vi "Start.vi"(6 "url (\"/mcp/server\")":string="/mcp/server", 8 "error in (no error)":errorcluster, 9 "HTTP Port (36987)":u16=36987, 10 "Description":string, 11 "Name":string) -> (0 "error out":errorcluster, 2 "MCP Events":T1, 3 "server id out":i32)   [LabVIEW 2020, in "MCP Server.lvlib"]
doc: "Creates a new MCP server. The URL will be:\nhttp://localhost:3687/mcp/server\nServer name and description will be passed on to the client and the LLM. Be aware that these cost you tokes. For detailled descriptions of the server (e.g. software manual) use resources instead. \nThis VI returns user events for different events that can happen inside the server. Make sure to listen to the error event to catch any runtime errors. Use the onRpc event to receive every request that is sent from a client to the server.\n\nYour MCP Client config (e.g. claude_desktop_config.json) should look like this:\n{\n \"mcpServers\": {\n \"My Cool Server Display-Name\": {\n \"command\": \"npx\",\n \"args\": [\n \"mcp-remote\",\n \"http://127.0.0.1:36987/mcp/server\"\n ],\n \"env\": {\n \"YOUR_API_KEY\": \"<YOUR_SECRET_KEY>\",\n \"MY_PARAM\": \"Your custom Parameter\"\n }\n }\n }\n}"
uses:
  MCP Server.lvlib
  User Events.ctl
  onRpc.ctl
  Server Data.ctl
  <vilib>/IlluminatedG/IG HTTP Server/HTTP Server/server/Server.lvclass
  Tool Data.ctl
  Input Parameter.ctl
  Output Parameter.ctl
  Logging.ctl
  Prompt Data.ctl
  Prompt Argument.ctl
  resource data.ctl
  MCP Handler/MCP Handler.lvclass
  C:/Program Files/National Instruments/LabVIEW 2026/vi.lib/IlluminatedG/IG HTTP Server/HTTP Server/Handler/Handler.lvclass
  <vilib>/IlluminatedG/IG HTTP Server/HTTP Server/Server/Add Connection Handler.vi
  <vilib>/IlluminatedG/IG HTTP Server/HTTP Server/Server/Add Request Handler.vi
  <vilib>/IlluminatedG/IG HTTP Server/HTTP Server/Server/Add Route Handler.vi
  <vilib>/IlluminatedG/IG HTTP Server/HTTP Server/Server/Add Controller Handler.vi
  <vilib>/IlluminatedG/IG HTTP Server/HTTP Server/Server/Add Controller.vi
  <vilib>/IlluminatedG/IG HTTP Server/HTTP Server/Server/Add Response Handler.vi
  <vilib>/IlluminatedG/IG HTTP Server/HTTP Server/Server/Add Complete Handler.vi
  <vilib>/IlluminatedG/IG HTTP Server/HTTP Server/Server/Add Exception Handler.vi
  <vilib>/IlluminatedG/IG HTTP Server/HTTP Server/Connection Handler/Connection Handler.lvclass
  <vilib>/IlluminatedG/IG HTTP Server/HTTP Server/Request Handler/Request Handler.lvclass
  <vilib>/IlluminatedG/IG HTTP Server/HTTP Server/Route Handler/Route Handler.lvclass
  <vilib>/IlluminatedG/IG HTTP Server/HTTP Server/Controller Handler/Controller Handler.lvclass
  <vilib>/IlluminatedG/IG HTTP Server/HTTP Server/Controller/Controller.lvclass
  <vilib>/IlluminatedG/IG HTTP Server/HTTP Server/Response Handler/Response Handler.lvclass
  <vilib>/IlluminatedG/IG HTTP Server/HTTP Server/Complete Handler/Complete Handler.lvclass
  <vilib>/IlluminatedG/IG HTTP Server/HTTP Server/Exception Handler/Exception Handler.lvclass
  <vilib>/IlluminatedG/IG HTTP Server/HTTP Server/Handler/Handler.lvclass
panel:
  out "server url":string
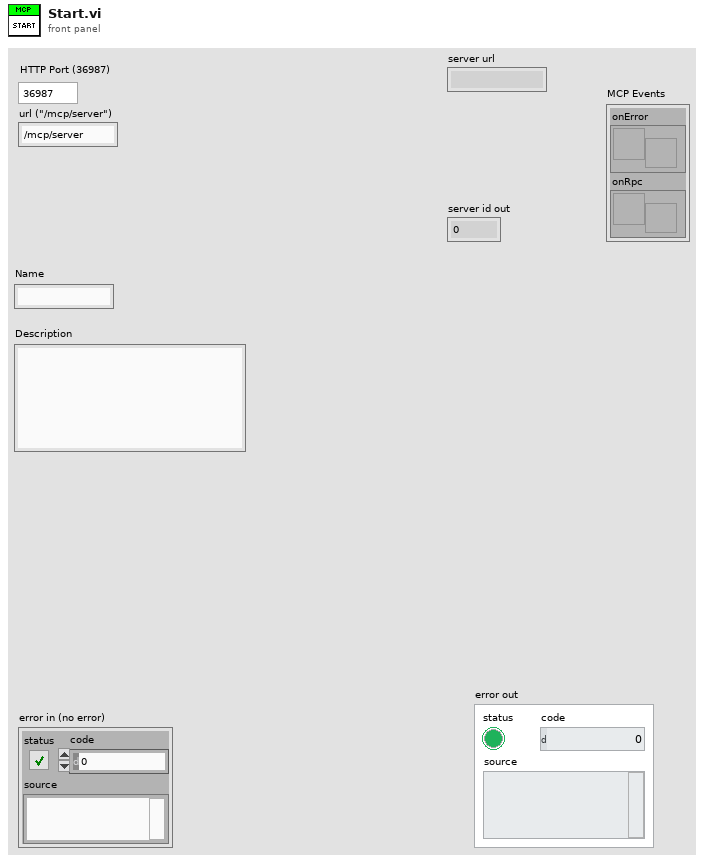
[diagram p1: front panel]
types:
  T1 = typedef "MCP Server.lvlib/User Events.ctl" = cluster{"onError":refnum<user-event>, "onRpc":refnum<user-event>}
  T2 = enum16{"Get", "GetAll", "Add", "Remove", "Clear"}
  T3 = typedef "MCP Server.lvlib/Server Data.ctl" = cluster{"Name":string, "Description":string, "Tools":T4[], "Parameters":string[][], "Logging Info":T7, "User Events":T1, "Prompts":T8[], "resources":T10[], "HTTP Server":refnum<class "Server.lvclass">}
  T4 = typedef "MCP Server.lvlib/Tool Data.ctl" = cluster{"Name":string, "Description":string, "Ignored":string[], "inputs":T5[], "outputs":T6[], "VI Refnum":refnum<vi>}
  T5 = typedef "MCP Server.lvlib/Input Parameter.ctl" = cluster{"name":string, "type":string, "description":string, "required":bool, "raw name":string}
  T6 = typedef "MCP Server.lvlib/Output Parameter.ctl" = cluster{"name":string, "description":string, "type":string, "raw name":string}
  T7 = typedef "MCP Server.lvlib/Logging.ctl" = cluster{"Log":string[], "Max Length":i32}
  T8 = typedef "MCP Server.lvlib/Prompt Data.ctl" = cluster{"name":string, "description":string, "arguments":T9[], "return terminal name":string, "results description":string, "VI Refnum":refnum<vi>}
  T9 = typedef "MCP Server.lvlib/Prompt Argument.ctl" = cluster{"name":string, "description":string, "required":bool, "raw_name":string}
  T10 = typedef "MCP Server.lvlib/resource data.ctl" = cluster{"uri":string, "name":string, "description":string, "mimeType":string, "file path":path}
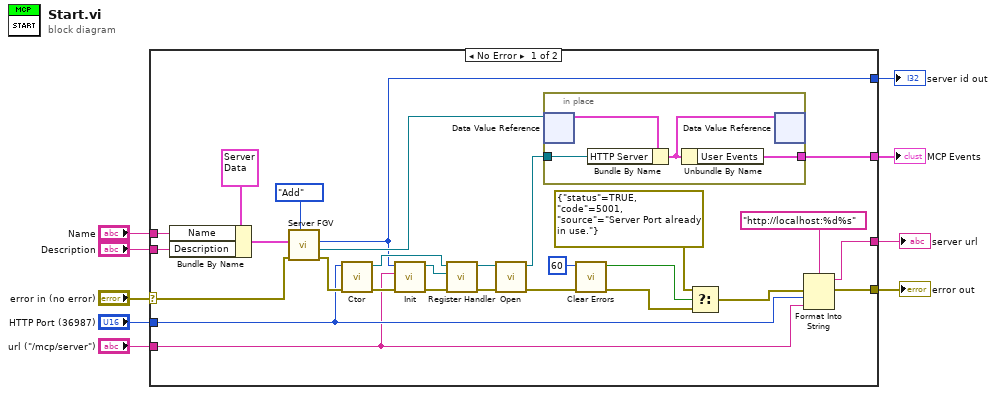
[diagram p0: block diagram]
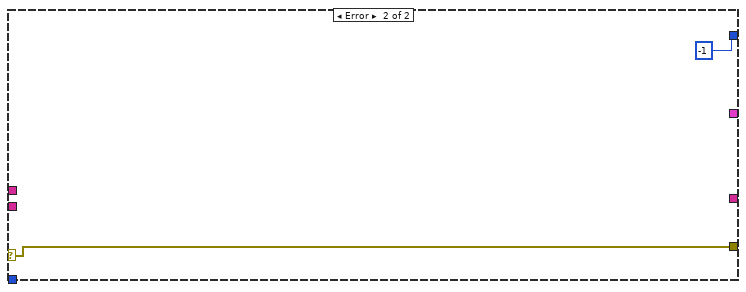
[diagram p2: hidden frame]
diagram:
  n1 = case shown="No Error" "error in (no error)" {
    selector: "error in (no error)" -> [w15 w43]
    tunnel: "Name" -> [w36 _]
    tunnel: "Description" -> [w35 _]
    tunnel: [w31 _] -> w7
    tunnel: [w25 -1 ("new id")] -> w6
    tunnel: "HTTP Port (36987)" -> [w20 _]
    tunnel: "url (\"/mcp/server\")" -> [w19 _]
    tunnel: [w17 w43] -> w3
    tunnel: [w16 _] -> w2
    frame No Error {
      n2 = Bundle By Name(cluster=T3 {"Name"="", "Description"="", "Tools"=[], "Parameters"=[], "Logging Info"={"Log"=[], "Max Length"=0}, "User Events"={"onError"=refnum, "onRpc"=refnum}, "Prompts"=[], "resources"=[], "HTTP Server"=refnum} ("New Server"), "Name"=w36, "Description"=w35) -> (w33:T3)
      n3 = call "Server FGV.vi"("Mode"=T2."Add", "error in"=w15, "New Server"=w33) -> ("error out"=w27:errorcluster, "server reference"=w32:refnum<data-value>, "new id"=w25:i32)  [unwired: 4 in, 2 out]
      n4 = call <vilib>:"Ctor.vi"("error in (no error)"=w27, "HTTP Port (80)"=w20) -> ("error out"=w23:errorcluster, "Server out"=w30:refnum<class "Server.lvclass">)  [unwired: 8 in]
      n5 = call "Init.vi"("error in (no error)"=w23, "url (\"/mcp/server\")"=w19, "id"=w25) -> ("error out"=w22:errorcluster, "MCP Handler out"=w24:refnum<class "MCP Handler.lvclass">)  [unwired: 7 in]
      n6 = call <vilib>:"Register Handler.vi"("error in (no error)"=w22, "Handler"=w24, "Server in"=w30) -> ("error out"=w28:errorcluster, "Server out"=w29:refnum<class "Server.lvclass">)  [unwired: 7 in]
      n7 = call <vilib>:"Open.vi"("error in (no error)"=w28, "Server in"=w29) -> ("error out"=w18:errorcluster, "Server out"=w26:refnum<class "Server.lvclass">)  [unwired: 8 in]
      n8 = in-place {
        in-place-border: [w40] -> w31
        in-place-border: w26 -> [w38]
        n9 = in-place-dvr #1(w32) -> (w41:T3)  [unwired: 1 out]
        n10 = Bundle By Name(cluster=w41, "HTTP Server"=w38) -> (w39:T3)
        n11 = Unbundle By Name(w39) -> ("User Events"=w40:T1)
        n12 = in-place-dvr #1(w39) -> ()  [unwired: 2 out]
      }
      n13 = call <vilib>:"Clear Errors.vi"("error in (no error)"=w18, "specific error code to clear (0: all)"=60) -> ("error out"=w14:errorcluster, "specific error cleared?"=w10:bool)  [unwired: 4 in]
      n14 = Select(t=errorcluster {"status"=TRUE, "code"=5001, "source"="Server Port already in use."} ("f"), s=w10, f=w14) -> (s? t:f=w12:errorcluster)
      n15 = Format Into String(format string="http://localhost:%d%s", error in=w12, w20, w19) -> (resulting string=w16:string, error out=w17:errorcluster)  [unwired: 1 in]
    }
    frame Error {
    }
  }
  "error out" <- w3
  "server id out" <- w6
  "MCP Events" <- w7
  "server url" <- w2
